vi "Maximum Packet Length.vi"() -> (0 "Max Packet Length":i32=1024)   [LabVIEW 2019, in "Network Messenger.lvlib"]
uses:
  <vilib>/gpm_packages/@cs/Network-interface/Source/Network Messenger/Network Messenger.lvlib
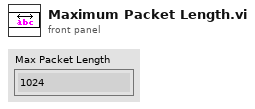
[diagram p1: front panel]
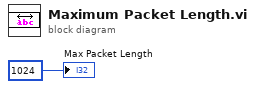
[diagram p0: block diagram]
diagram:
  "Max Packet Length" <- 1024 ("y")
